vi "Get DLL Path.vi"() -> (0 "DLL Path":path)   [LabVIEW 2013, in "Keyence LK-G5000.lvlib"]
uses:
  <instrlib>/Keyence LK-G5000/Keyence LK-G5000.lvlib
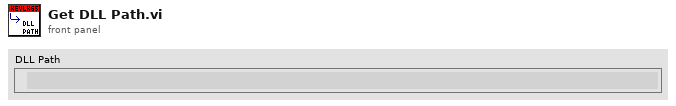
[diagram p1: front panel]
types:
  T1 = enum32{"invalid app kind", "Development System", "Run Time System", "Student Edition", "Embedded LabVIEW", "Evaluation", "Custom"}
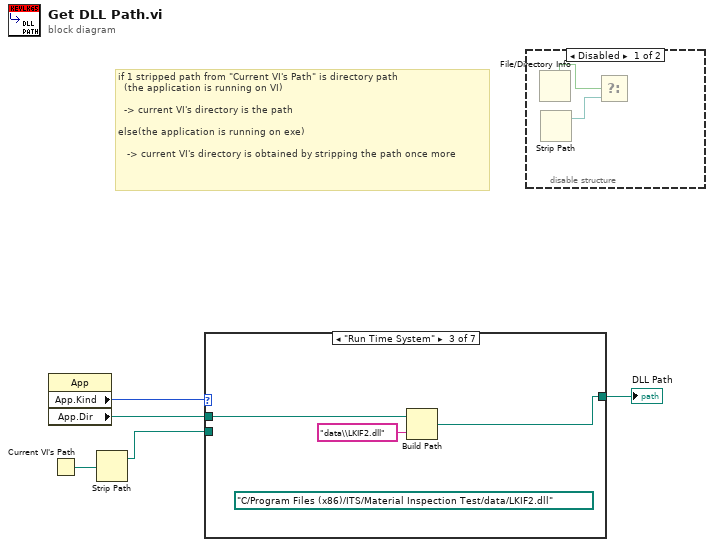
[diagram p0: block diagram]
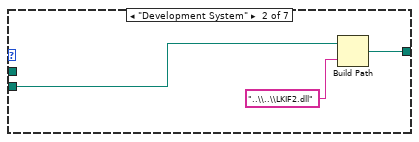
[diagram p4: hidden frame]
diagram:
  # "if 1 stripped path from \"Current VI's Path\" is directory path\n  (the application is running on VI)\n\n  -> current VI's directory is the path\n\nelse(the application is running on exe)\n\n　-> current VI's directory is obtained by stripping the path once more"
  n1 = property class="App"() -> ("App.Kind"=w5:T1, "App.Dir"=w2:path)  [unwired: 2 in, 2 out]
  n2 = Current VI's Path() -> (path=w4:path)
  n3 = Strip Path(path=w4) -> (stripped path=w3:path)  [unwired: 1 out]
  n4 = case shown="\"Run Time System\"" w5 {
    tunnel: [_ w6 w9 _ _ _ _] -> w1
    tunnel: w3 -> [_ w7 _ _ _ _ _]
    tunnel: w2 -> [_ _ w11 _ _ _ _]
    frame "invalid app kind", Default {
    }
    frame "Development System" {
      n5 = Build Path(base path=w7, name or relative path="..\\..\\LKIF2.dll" ("名前または相対パス")) -> (appended path=w6:path)
    }
    frame "Run Time System" {
      (unwired) path "C:/Program Files (x86)/ITS/Material Inspection Test/data/LKIF2.dll" ("stripped path")
      n6 = Build Path(base path=w11, name or relative path="data\\LKIF2.dll") -> (appended path=w9:path)
    }
    frame "Student Edition" {
    }
    frame "Embedded LabVIEW" {
    }
    frame "Evaluation" {
    }
    frame "Custom" {
    }
  }
  "DLL Path" <- w1
  n7 = disable-structure shown="Disabled" {
    frame Disabled {
      n8 = File/Directory Info() -> (directory=w13:bool)  [unwired: 2 in, 6 out]
      n9 = Strip Path() -> (stripped path=w12:path)  [unwired: 1 in, 1 out]
      n10 = Select(s=w13, f=w12) -> ()  [unwired: 1 in, 1 out]
    }
    frame Enabled {
    }
  }
